vi "File List Clear.vi"(11 "File List in":refnum<class "File List.lvclass">) -> (3 "File List out":refnum<class "File List.lvclass">)   [LabVIEW 2014, in "COSYLib.lvlib" / "File List.lvclass"]
uses:
  File List.lvclass
  File List.lvclass/File List.ctl
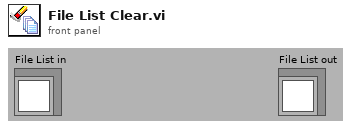
[diagram p1: front panel]
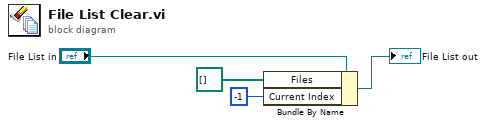
[diagram p0: block diagram]
diagram:
  n1 = Bundle By Name(cluster="File List in", "Files"=path[] [], "Current Index"=-1) -> (→"File List out":refnum<class "File List.lvclass">)
